vi "Mono.init.vi"(11 "Mono in":T1) -> (3 "Mono out":T1)   [LabVIEW 2022 SP3]
panel:
  out "reply":string
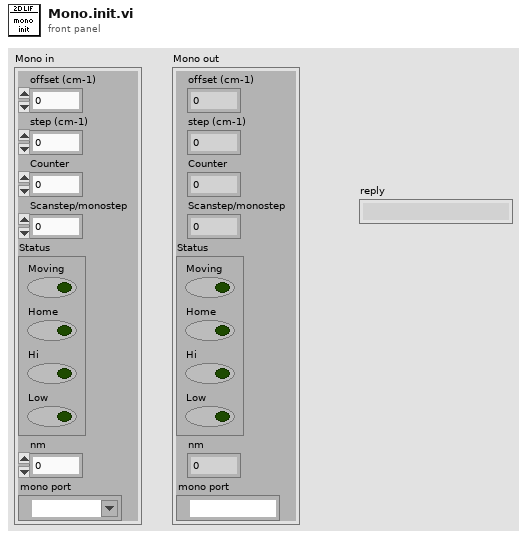
[diagram p1: front panel]
types:
  T1 = cluster{"offset (cm-1)":dbl, "step (cm-1)":dbl, "Counter":dbl, "Scanstep/monostep":i32, "Status":cluster{"Moving":bool, "Home":bool, "Hi":bool, "Low":bool}, "nm":dbl, "mono port":refnum<visa-resource-name>}
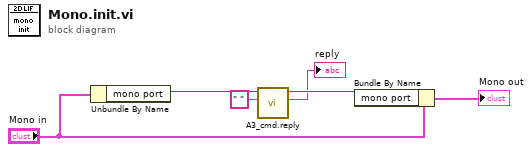
[diagram p0: block diagram]
diagram:
  n1 = Unbundle By Name("Mono in") -> ("mono port"=w3:refnum<visa-resource-name>)
  n2 = call "A3_cmd.reply.vi"("cmd"=" ", "VISA resource name"=w3) -> ("reply"=→"reply":string, "VISA resource name out"=w5:refnum<visa-resource-name>)  [unwired: 7 in, 1 out]
  n3 = Bundle By Name(cluster="Mono in", "mono port"=w5) -> (→"Mono out":T1)
